vi "svx_Orbit Image.vi"(6 "State":T2={"X Scale"={"Name"="Horizontal", "FString"="%#.2g", "Major Color"=16777238, "Minor Color"=16777216, "Scale Visible"=TRUE, " Label Visible"=TRUE, "Grid Style"=1}, "Y Scale"={"Name"="Vertical", "FString"="%#.2g", "Major Color"=16777238, "Minor Color"=16777216, "Scale Visible"=TRUE, " Label Visible"=TRUE, "Grid Style"=1}, "Plot"={"Point Style"=0, "Line Width"=0, "Line Style"=0, "Plot Color"=9727, "Point/fill"=0}, "Arrow/Crosshair Color"=9727, "Tacho Point Color"=16711680, "Container Bounds"={"Width"=563, "Height"=294}, "Axis Maximum"=10.0, "Probe Angles"={"Angle X"=0.0, "Angle Y"=1.5707963267948966}, "Background Color"=16777226, "Cursor"={"Cursor Point Style"=13, "Cursor Style"=4, "Cursor Line Width"=1, "Cursor Line Style"=0, "Cursor Color"=9727, "Cursor Name Visible"=TRUE, "Cursor Visible"=TRUE, "Cursor Position"={"X"=0.0, "Y"=0.0}, "Cursor Index"=0, "Cursor Lock"=FALSE}, "Elliptical Info"=[], "Legend Visible"=TRUE, "Scale Range Change"=refnum, "Strings[]"={"Custom pair name"=FALSE, "Row Strings []"=[], "Column Strings []"=[]}, "Index"=[{"pair index"=0, "order index"=0}], " Parents Tags"=[], "Children Tags"=[], "Open?"=[], "Label"="", "Legend Width"=120, "Pair Strings Changed?"=FALSE, "Size"=[], "Legend Background"=16777226, "Legend Font"=16777222, "Cursor Release"=refnum, "Autoscale"=TRUE, "Precession Direction"=[], "Item Width"=0, "User Pair Strings []"=[], "Users Order Strings []"=[], "Autoscale Once"=TRUE, "Property Write"=refnum} {"Index"."order index" min=0; "Index"."pair index" min=0; "Axis Maximum" min=0.0}, 7 "Orbit Plot":T1, 10 "Plot Area:Size":T4={"Width"=536, "Height"=536}, 11 "Picture In":picture) -> (3 "Picture Out":picture)   [LabVIEW 2017, in "SVX Orbit.xctl"]
uses:
  <vilib>/addons/_XControls/Orbit Plot/SVX Orbit.xctl
  <vilib>/Utility/miscctls.llb/LVBoundsTypeDef.ctl
  <vilib>/addons/_XControls/Orbit Plot/subVIs/svx_Orbit Internal State.ctl
  <vilib>/addons/_XControls/Orbit Plot/subVIs/svx_Orbit Bounds.ctl
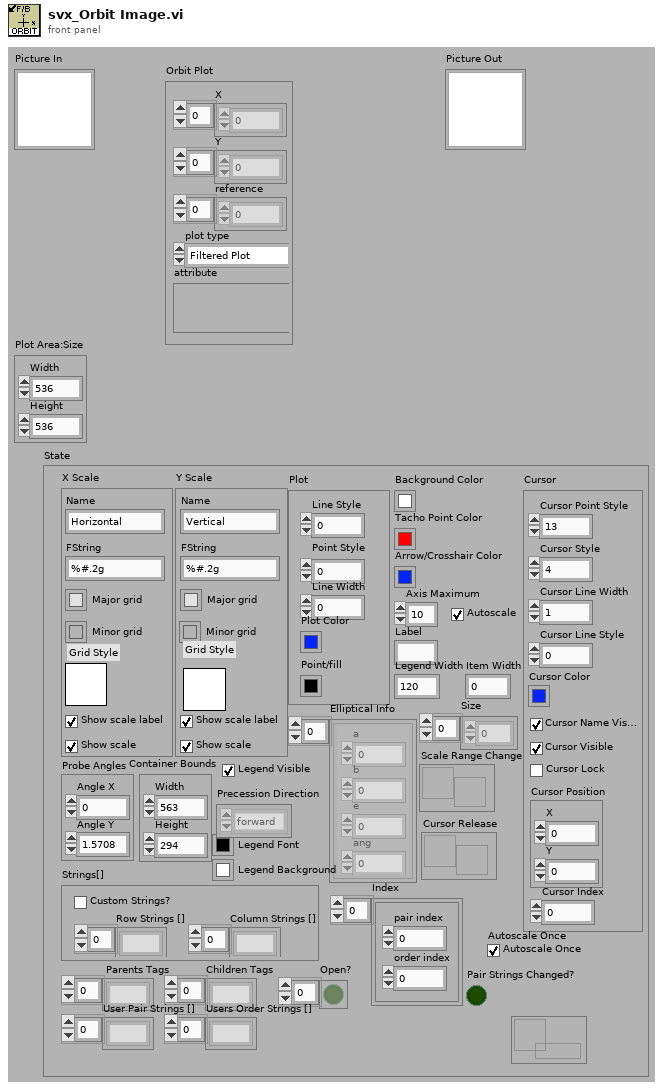
[diagram p1: front panel]
types:
  T1 = cluster{"X":dbl[], "Y":dbl[], "reference":dbl[], "plot type":enum16{"Filtered Plot", "Unfiltered Plot"}, "attribute":variant}
  T2 = typedef "SVX Orbit.xctl/svx_Orbit Internal State.ctl" = cluster{"X Scale":cluster{"Name":string, "FString":string, "Major Color":u32, "Minor Color":u32, "Scale Visible":bool, " Label Visible":bool, "Grid Style":u16}, "Y Scale":cluster{"Name":string, "FString":string, "Major Color":u32, "Minor Color":u32, "Scale Visible":bool, " Label Visible":bool, "Grid Style":u16}, "Plot":cluster{"Point Style":u8, "Line Width":u8, "Line Style":u8, "Plot Color":u32, "Point/fill":u32}, "Arrow/Crosshair Color":u32, "Tacho Point Color":u32, "Container Bounds":T3, "Axis Maximum":dbl, "Probe Angles":cluster{"Angle X":dbl, "Angle Y":dbl}, "Background Color":u32, "Cursor":cluster{"Cursor Point Style":u8, "Cursor Style":u8, "Cursor Line Width":u8, "Cursor Line Style":u8, "Cursor Color":u32, "Cursor Name Visible":bool, "Cursor Visible":bool, "Cursor Position":cluster{"X":dbl, "Y":dbl}, "Cursor Index":i32, "Cursor Lock":bool}, "Elliptical Info":cluster{"a":dbl, "b":dbl, "e":dbl, "ang":dbl}[], "Legend Visible":bool, "Scale Range Change":refnum<user-event>, "Strings[]":cluster{"Custom pair name":bool, "Row Strings []":string[], "Column Strings []":string[]}, "Index":cluster{"pair index":i32, "order index":i32}[], " Parents Tags":string[], "Children Tags":string[], "Open?":bool[], "Label":string, "Legend Width":u32, "Pair Strings Changed?":bool, "Size":i32[], "Legend Background":u32, "Legend Font":u32, "Cursor Release":refnum<user-event>, "Autoscale":bool, "Precession Direction":enum16{"forward", "backward"}[], "Item Width":u32, "User Pair Strings []":string[], "Users Order Strings []":string[], "Autoscale Once":bool, "Property Write":refnum<queue>}
  T3 = typedef "SVX Orbit.xctl/svx_Orbit Bounds.ctl" = cluster{"Width":u32, "Height":u32}
  T4 = typedef "LVBoundsTypeDef.ctl" = cluster{"Width":u32, "Height":u32}
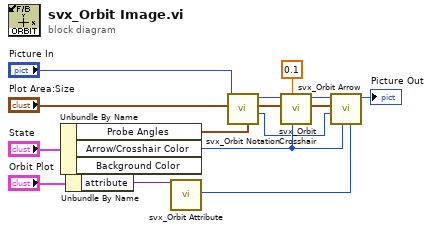
[diagram p0: block diagram]
diagram:
  n1 = Unbundle By Name("State") -> ("Probe Angles"=w10:cluster{"Angle X":dbl, "Angle Y":dbl}, "Arrow/Crosshair Color"=w8:u32)  [unwired: 1 out]
  n2 = Unbundle By Name("Orbit Plot") -> ("attribute"=w3:variant)
  n3 = call <vilib>:"svx_Orbit Attribute.vi"("attribute"=w3) -> ("rotating direction"=w5:u16)  [unwired: 13 in, 5 out]
  n4 = call <vilib>:"svx_Orbit Notation.vi"("probe angles"=w10, "Plot Area:Size"="Plot Area:Size", "Picture in"="Picture In") -> ("text max size"=w2:i16, "Plot Area:Size out"=w13:T4, "Picture out"=w11:picture)  [unwired: 6 in]
  n5 = call <vilib>:"svx_Orbit Crosshair.vi"("crosshair color"=w8, "crosshair size %"=0.1, "Plot Area:Size in"=w13, "Picture in"=w11) -> ("Plot Area:Size out"=w6:T4, "Picture out"=w1:picture)  [unwired: 6 in]
  n6 = call <vilib>:"svx_Orbit Arrow.vi"("shaft rotating direction"=w5, "color"=w8, "text max size"=w2, "Plot Area:Size"=w6, "Picture in"=w1) -> ("new picture"=→"Picture Out":picture)  [unwired: 5 in, 1 out]
